vi "INSTRU_FINAL_PROY.vi"() -> ()   [LabVIEW 2021]
uses:
  <vilib>/userDefined/High Color/IMAQdx.ctl
  <vilib>/Instr/_visa.llb/VISA Configure Serial Port (Instr).vi
  <vilib>/vision/driver/NI_Vision_Acquisition_Software.lvlib
  <vilib>/vision/NI_Vision_Development_Module.lvlib
panel:
  in  "PARO DE EMERGENCIA":bool
  in  "PUERTO COM ARDUINO":refnum<visa-resource-name>
  out "ROJO":bool
  out "VERDE":bool
  out "AZUL":bool
  in  "SENSIBILIDAD DE CAMARA":u32(ring) items=["Low", "Medium", "High"]
  in  "PUERTO COM CAMARA":T1
  out "Image":T2(plugin-control)
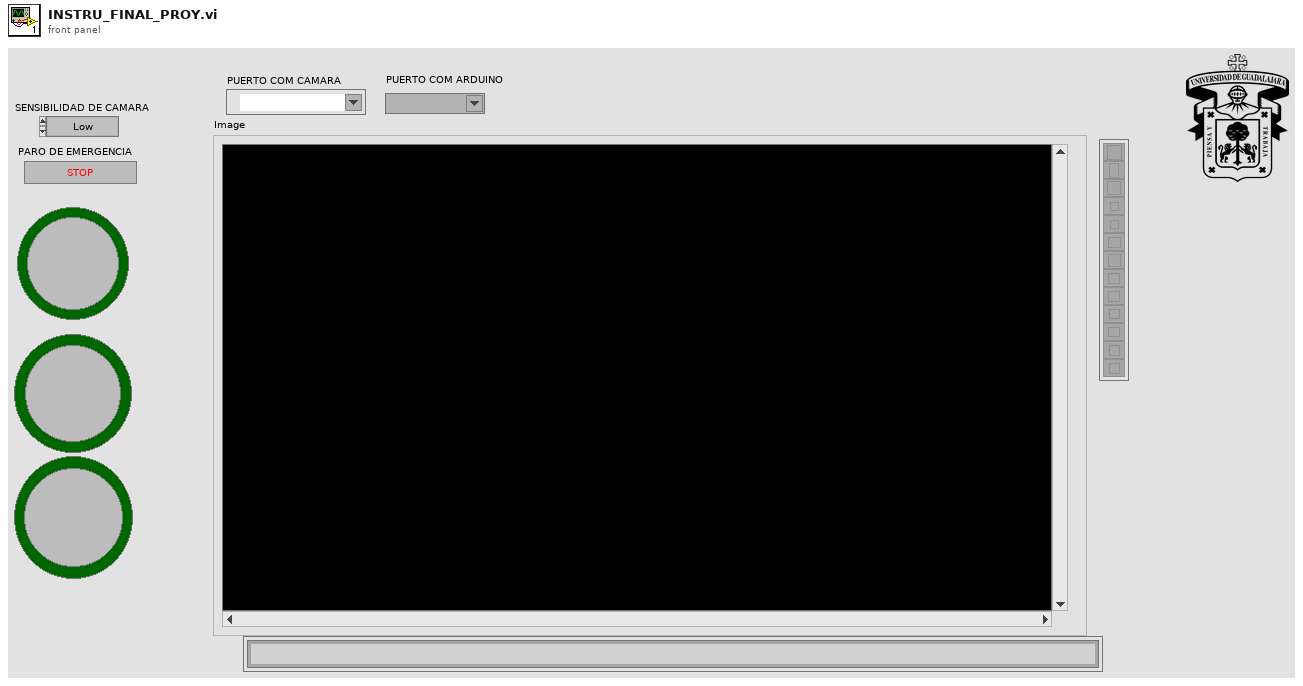
[diagram p1: front panel]
types:
  T1 = typedef "IMAQdx.ctl" = refnum<k21>
  T2 = typedef "IMAQ Image.ctl" = refnum<image>
  T3 = cluster{"Global Rectangle":i32[], "Contours":cluster{"Contour Type":u32, "ROI Type":u32, "Points":i32[]}[]}
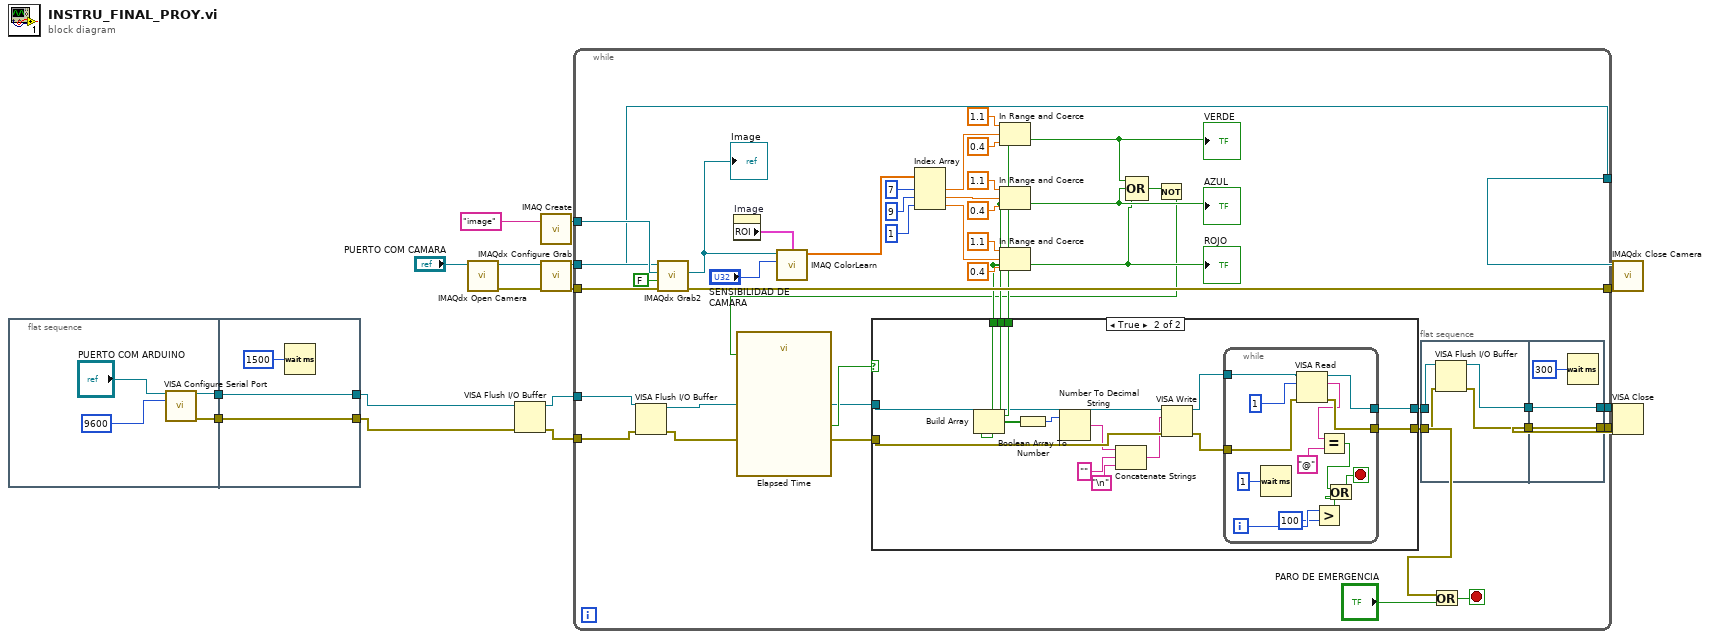
[diagram p0: block diagram]
diagram:
  n1 = flat-sequence {
    tunnel: [w20] -> w2
    tunnel: [w19] -> w1
    tunnel: [w23] -> w7
    tunnel: [w24] -> w8
    tunnel: w2 -> [w24]
    tunnel: w1 -> [w23]
    frame #0 {
      n2 = call-poly "VISA Configure Serial Port"("VISA resource name"="PUERTO COM ARDUINO", "baud rate (9600)"=u32 9600) -> ("VISA resource name out"=w19:refnum<visa-resource-name>, "error out"=w20:errorcluster)  [unwired: 12 in]
    }
    frame #1 {
      n3 = Wait (ms)(milliseconds to wait=u32 1500) -> ()  [unwired: 1 out]
    }
  }
  n4 = call <vilib>:"IMAQdx Open Camera.vi"("Session In"="PUERTO COM CAMARA") -> ("error out"=w16:errorcluster, "Session Out"=w17:T1)  [unwired: 9 in]
  n5 = VISA Flush I/O Buffer(VISA resource name=w7, error in (no error)=w8) -> (VISA resource name out=w6:refnum<visa-resource-name>, error out=w5:errorcluster)  [unwired: 1 in]
  n6 = call "IMAQ Create"("Image Name"="image") -> ("New Image"=w14:T2)  [unwired: 4 in, 1 out]
  n7 = call <vilib>:"IMAQdx Configure Grab.vi"("error in"=w16, "Session In"=w17) -> ("error out"=w12:errorcluster, "Session Out"=w13:T1)  [unwired: 8 in]
  n8 = while {
    tunnel: w14 -> [w64]
    tunnel: w13 -> [w63]
    tunnel: w12 -> [w62]
    tunnel: [w61] -> w11
    tunnel: [w45] -> w10
    tunnel: w6 -> [w31]
    tunnel: w5 -> [w29]
    tunnel: [w33] -> w4
    tunnel: [w32] -> w3
    stop <- w43 stop-if-true
    n9 = VISA Flush I/O Buffer(VISA resource name=w31, error in (no error)=w29) -> (VISA resource name out=w30:refnum<visa-resource-name>, error out=w28:errorcluster)  [unwired: 1 in]
    n10 = call <vilib>:"IMAQdx Grab2.vi"("error in"=w62, "Wait for Next Buffer? (Yes)"=FALSE, "Image In"=w64, "Session In"=w63) -> ("error out"=w45:errorcluster, "Image Out"=w58:T2, "Session Out"=w61:T1)  [unwired: 4 in, 1 out]
    "Image" <- w58
    n11 = property on="Image" class="ImageControl"() -> ("ROI"=w60:T3)  [unwired: 2 in, 2 out]
    n12 = call "IMAQ ColorLearn"("ROI Descriptor"=w60, "Image"=w58, "Color Sensitivity"="SENSIBILIDAD DE CAMARA") -> ("Color Spectrum"=w59:dbl[])  [unwired: 5 in, 1 out]
    n13 = Index Array(array=w59, index #1=7 ("index"), index #2=9 ("index"), index #3=1 ("index")) -> (element #1=w54:dbl, element #2=w49:dbl, element #3=w48:dbl)
    n14 = In Range and Coerce(upper limit=1.1, x=w54, lower limit=0.4) -> (In Range?=w41:bool)  [unwired: 1 out]
    "VERDE" <- w41
    n15 = In Range and Coerce(upper limit=1.1, x=w49, lower limit=0.4) -> (In Range?=w40:bool)  [unwired: 1 out]
    "AZUL" <- w40
    n16 = In Range and Coerce(upper limit=1.1, x=w48, lower limit=0.4) -> (In Range?=w39:bool)  [unwired: 1 out]
    "ROJO" <- w39
    n17 = Compound Arithmetic op=OR(w41, w40, w39) -> (w37:bool)
    n18 = Not(x=w37) -> (.not. x?=w36:bool)
    n19 = call "Elapsed Time"("Reset"=w36) -> ("Time has Elapsed"=w42:bool)  [unwired: 11 in, 7 out]
    n20 = case shown="True" w42 {
      tunnel: w41 -> [_ w87]
      tunnel: w40 -> [_ w86]
      tunnel: w39 -> [_ w85]
      tunnel: [w73 w75] -> w35
      tunnel: w30 -> [w73 w83]
      tunnel: w28 -> [w72 w82]
      tunnel: [w72 w74] -> w34
      frame False {
      }
      frame True {
        n21 = Build Array(w87, w86, w85) -> (w84:bool[])
        n22 = Boolean Array To Number(Boolean array=w84) -> (number=w88:u32)
        n23 = Number To Decimal String(number=w88) -> (decimal integer string=w81:string)  [unwired: 1 in]
        n24 = Concatenate Strings(w81, "" ("string"), "\n") -> (w80:string)
        n25 = VISA Write(VISA resource name=w83, write buffer=w80, error in (no error)=w82) -> (VISA resource name out=w77:refnum<visa-resource-name>, error out=w76:errorcluster)  [unwired: 1 out]
        n26 = while {
          tunnel: w77 -> [w100]
          tunnel: w76 -> [w99]
          tunnel: [w98] -> w75
          tunnel: [w97] -> w74
          i -> [w94]
          stop <- w90 stop-if-true
          n27 = Wait (ms)(milliseconds to wait=u32 1) -> ()  [unwired: 1 out]
          n28 = VISA Read(VISA resource name=w100, byte count=1 ("index"), error in (no error)=w99) -> (VISA resource name out=w98:refnum<visa-resource-name>, read buffer=w96:string, error out=w97:errorcluster)  [unwired: 1 out]
          n29 = Greater?(x=w94, y=100) -> (0:w92:bool)
          n30 = Equal?(x=w96, y="@" ("string")) -> (x = y?=w91:bool)
          n31 = Or(x=w91, y=w92) -> (x .or. y?=w90:bool)
        }
      }
    }
    n32 = flat-sequence {
      tunnel: w35 -> [w68]
      tunnel: w34 -> [w67]
      tunnel: [w66] -> w26
      tunnel: [w65] -> w25
      tunnel: [w70] -> w32
      tunnel: [w71] -> w33
      tunnel: w26 -> [w71]
      tunnel: w25 -> [w70]
      frame #0 {
        n33 = VISA Flush I/O Buffer(VISA resource name=w68, error in (no error)=w67) -> (VISA resource name out=w66:refnum<visa-resource-name>, error out=w65:errorcluster)  [unwired: 1 in]
      }
      frame #1 {
        n34 = Wait (ms)(milliseconds to wait=u32 300) -> ()  [unwired: 1 out]
      }
    }
    n35 = Or(x=w34, y="PARO DE EMERGENCIA") -> (x .or. y?=w43:bool)
  }
  n36 = call <vilib>:"IMAQdx Close Camera.vi"("error in"=w10, "Session In"=w11) -> ()  [unwired: 9 in, 1 out]
  n37 = VISA Close(VISA resource name=w4, error in (no error)=w3) -> ()  [unwired: 1 out]
